vi "ClassProvidor_GoopOptionsDialog.vi"(8 "error in (no error)":errorcluster) -> (0 "error out":errorcluster)   [LabVIEW 2020]
uses:
  <resource>/Framework/Providers/Open_GDS/SubVIs/GOOP_HelpButton.ctl
  <resource>/Framework/Providers/Open_GDS/ClassProviders/Provider_EndevoGOOP300/EndevoProviderName.ctl
  <resource>/Framework/Providers/Open_GDS/ClassProviders/Provider_EndevoGOOP400/EndevoG4ProviderName.ctl
panel:
  in  "_InstallNewClassProvider":bool
  in  "_RemoveClassProvider":bool
  in  "_HelpGoopOption":T1
  in  "_AddClassProvider":bool
  out "Tab":enum32{"Select", "Add"}(tab)
  in  "_CurrentClassProvider":u16(ring) caption="Current Class provider to use:" items=["EndevoGOOP300", "Endevo LabVIEW Native", "EndevoGOOP400"]
  in  "_ConfigureCurrentClassProvider":bool
  out "ProductPicture":picture
  in  "_ProviderClassReaderPath":path caption="Provider Class Reader Path"
  in  "_ProviderClassWriterPath":path caption="Provider Class Writer Path"
  in  "_ProviderName":string caption="ProviderName"
  in  "_Cancel":bool
  in  "_OK":bool
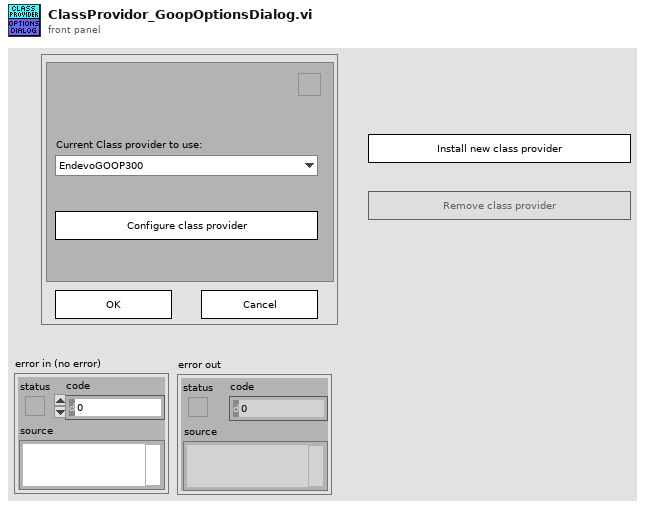
[diagram p1: front panel]
types:
  T1 = typedef "GOOP_HelpButton.ctl" = bool
  T2 = typedef "EndevoG4ProviderName.ctl" = enum16{"EndevoGOOP400"}
  T3 = typedef "EndevoProviderName.ctl" = enum16{"EndevoGOOP300"}
  T4 = cluster{"ClassProviders":string[], "Path":path, "ClassConfig":path}
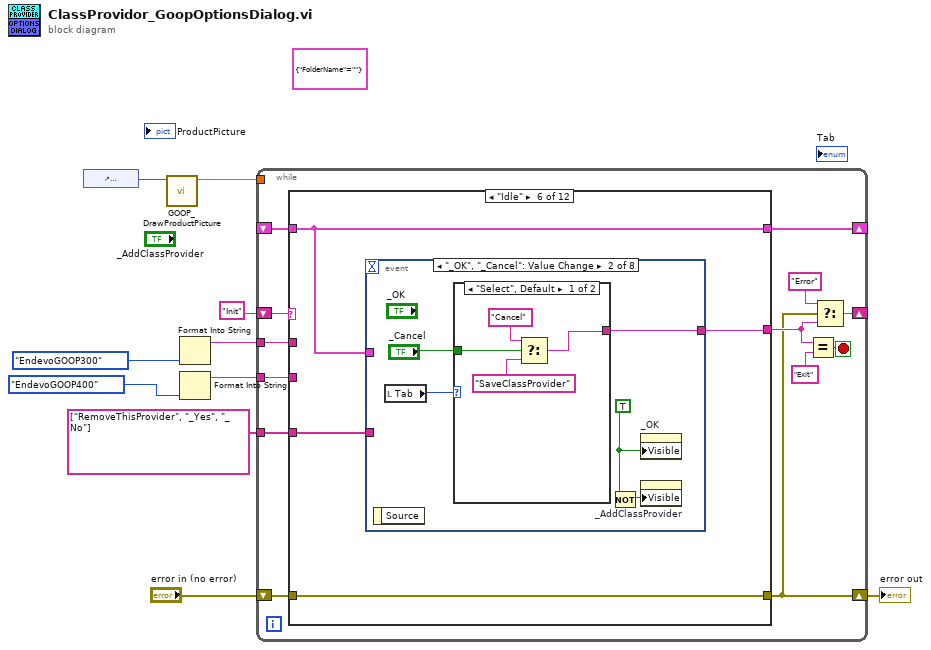
[diagram p0: block diagram]
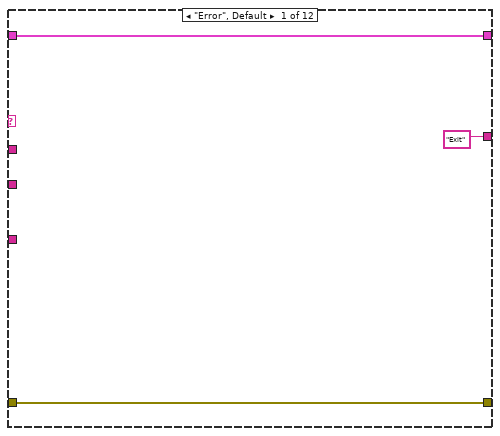
[diagram p2: hidden frame]
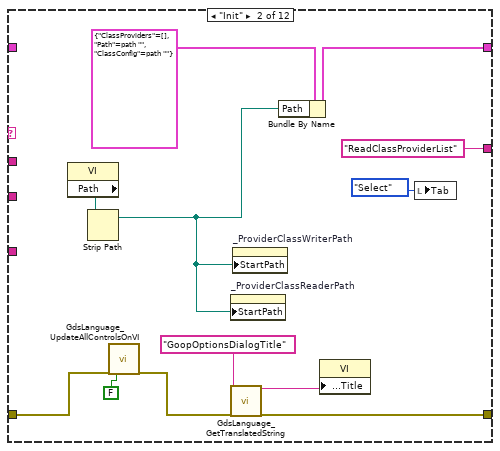
[diagram p3: hidden frame]
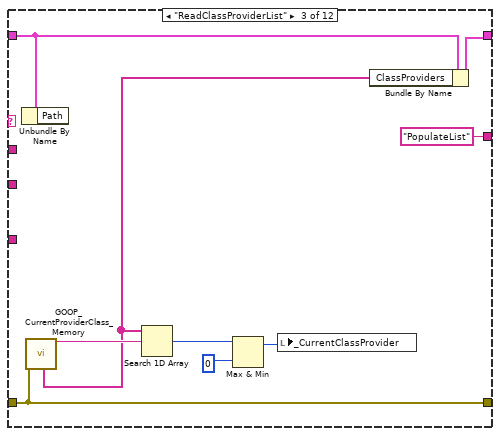
[diagram p4: hidden frame]
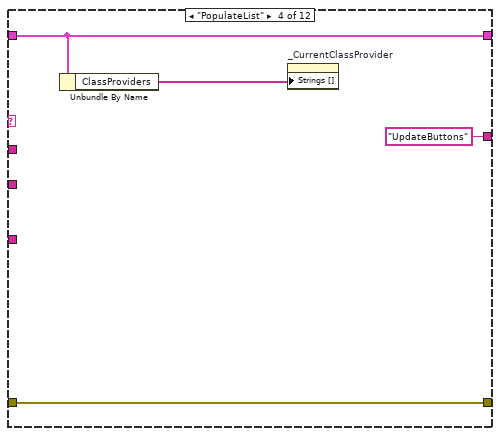
[diagram p5: hidden frame]
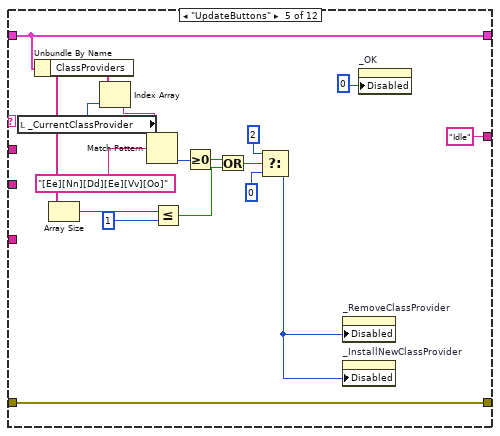
[diagram p6: hidden frame]
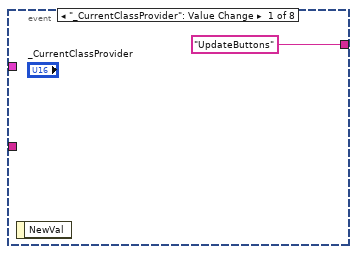
[diagram p7: hidden frame]
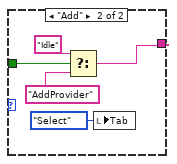
[diagram p8: hidden frame]
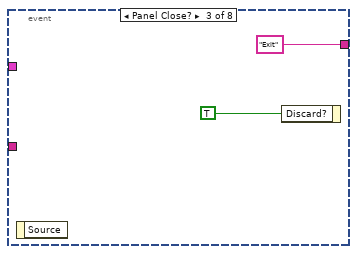
[diagram p9: hidden frame]
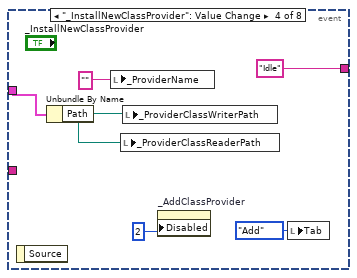
[diagram p10: hidden frame]
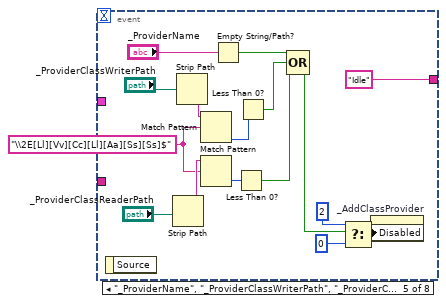
[diagram p11: hidden frame]
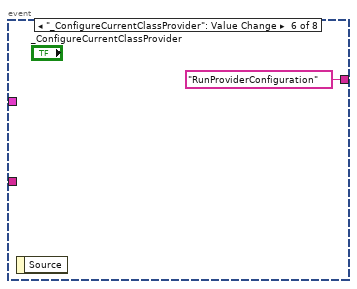
[diagram p12: hidden frame]
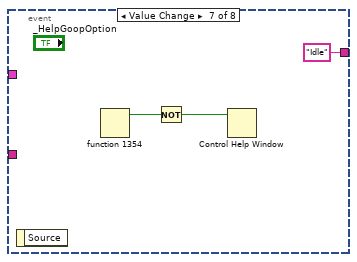
[diagram p13: hidden frame]
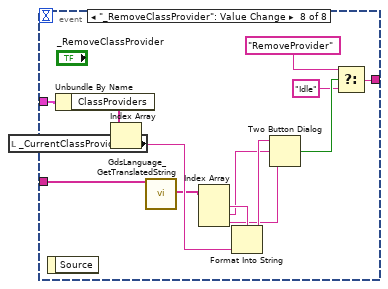
[diagram p14: hidden frame]
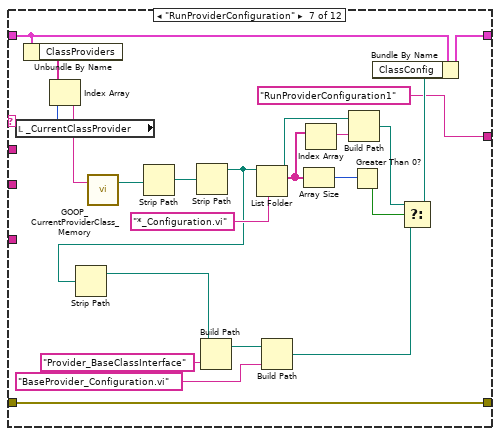
[diagram p15: hidden frame]
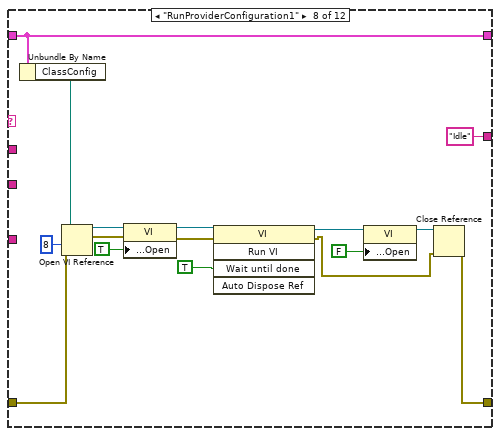
[diagram p16: hidden frame]
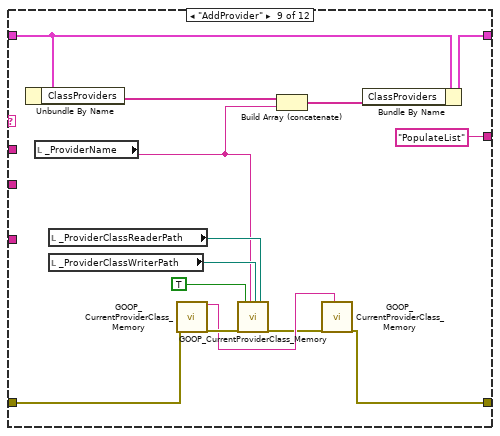
[diagram p17: hidden frame]
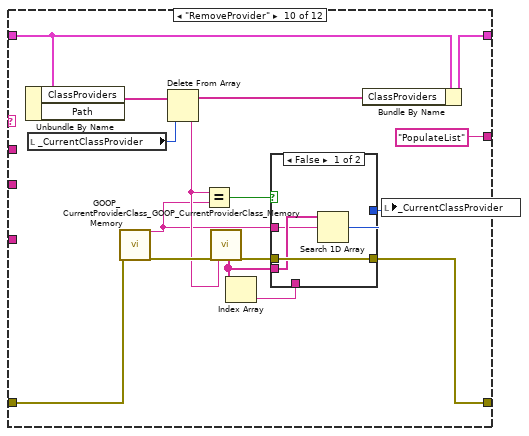
[diagram p18: hidden frame]
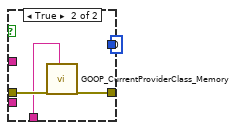
[diagram p19: hidden frame]
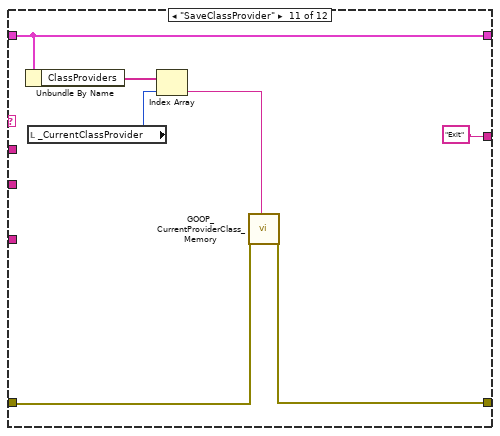
[diagram p20: hidden frame]
diagram:
  (unwired) cluster{"FolderName":string} {"FolderName"=""}
  n1 = control-ref of="ProductPicture"() -> (w2:refnum<vi>)
  n2 = call <resource>:"GOOP_DrawProductPicture.vi"("ProductPictureControl"=w2) -> ("Zoom Factor"=w1:sgl)  [unwired: 10 in]
  n3 = Format Into String(EndevoProviderName."EndevoGOOP300" ("ProviderName")) -> (resulting string=w4:string)  [unwired: 3 in, 1 out]
  n4 = Format Into String(EndevoG4ProviderName."EndevoGOOP400" ("ProviderName")) -> (resulting string=w3:string)  [unwired: 3 in, 1 out]
  n5 = while {
    shift-right: [w16] -> w8
    shift-left: "error in (no error)" -> [w23]
    shift-right: [w21] -> _
    shift-left: "Init" -> [w22]
    shift-right: [w15] -> _
    shift-left: _ -> [w14]
    tunnel: string[] ["RemoveThisProvider", "_Yes", "_No"] -> [w13]
    tunnel: w4 -> [w12]
    tunnel: w3 -> [w11]
    tunnel: w1 -> [_]
    stop <- w20 stop-if-true
    n6 = case shown="\"Idle\"" w22 {
      tunnel: w23 -> [w26 w31 w45 w48 w56 w71 w149 w167 w173 w192 w211 w214]
      tunnel: [w26 w28 w45 w48 w56 w71 w149 w165 w169 w186 w210 w214] -> w16
      tunnel: ["Exit" "ReadClassProviderList" "PopulateList" "UpdateButtons" "Idle" w72 "RunProviderConfiguration1" "Idle" ("f") "PopulateList" "PopulateList" "Exit" "Exit"] -> w17
      tunnel: [w24 w35 w46 w50 w58 w70 w147 w164 w182 w198 w213 w216] -> w15
      tunnel: w14 -> [w24 _ w42 w50 w58 w70 w148 w164 w181 w197 w213 w216]
      tunnel: w13 -> [_ _ _ _ _ w69 _ _ _ _ _ _]
      tunnel: w12 -> [_ _ _ _ _ _ _ _ _ _ _ _]
      tunnel: w11 -> [_ _ _ _ _ _ _ _ _ _ _ _]
      frame "Error", Default {
      }
      frame "Init" {
        n7 = property class="VI"() -> ("Path"=w34:path)  [unwired: 2 in, 2 out]
        n8 = Strip Path(path=w34) -> (stripped path=w33:path)  [unwired: 1 out]
        n9 = call <resource>:"GdsLanguage_UpdateAllControlsOnVI.vi"("error in (no error)"=w31, "CreateLanguageFile(Use this to create a languageFile)"=FALSE) -> ("error out"=w30:errorcluster)  [unwired: 16 in, 1 out]
        n10 = property on="_ProviderClassReaderPath" class="Path"("StartPath"=w33) -> ()  [unwired: 2 in, 2 out]
        n11 = call <resource>:"GdsLanguage_GetTranslatedString.vi"("StringID(s)"="GoopOptionsDialogTitle", "error in (no error)"=w30) -> ("FirstStringOut"=w27:string, "error out"=w28:errorcluster)  [unwired: 14 in, 2 out]
        n12 = property on="_ProviderClassWriterPath" class="Path"("StartPath"=w33) -> ()  [unwired: 2 in, 2 out]
        n13 = Bundle By Name(cluster=T4 {"ClassProviders"=[], "Path"=path "", "ClassConfig"=path ""}, "Path"=w33) -> (w35:T4)
        n14 = property class="VI"("Front Panel.Title"=w27) -> ()  [unwired: 2 in, 2 out]
        n15 = local write "Tab"(enum32{"Select", "Add"}."Select" ("Tab")) -> ()
      }
      frame "ReadClassProviderList" {
        n16 = Unbundle By Name(w42) -> ()  [unwired: 1 out]
        n17 = call <resource>:"GOOP_CurrentProviderClass_Memory.vi"("error in (no error)"=w45) -> ("AllClassProviders"=w43:string[], "ClassProviderName"=w44:string)  [unwired: 14 in, 3 out]
        n18 = Search 1D Array(1D array=w43, element=w44) -> (index of element=w41:i32)  [unwired: 1 in]
        n19 = Max & Min(x=w41, y=0 ("lower limit")) -> (max(x,y)=w39:i32)  [unwired: 1 out]
        n20 = local write "_CurrentClassProvider"(w39) -> ()
        n21 = Bundle By Name(cluster=w42, "ClassProviders"=w43) -> (w46:T4)
      }
      frame "PopulateList" {
        n22 = Unbundle By Name(w50) -> ("ClassProviders"=w49:string[])
        n23 = property on="_CurrentClassProvider" class="Ring (strict)"("Strings []"=w49) -> ()  [unwired: 2 in, 2 out]
      }
      frame "UpdateButtons" {
        n24 = local read "_CurrentClassProvider"() -> (w54:u16)
        n25 = Unbundle By Name(w58) -> ("ClassProviders"=w67:string[])
        n26 = Array Size(array=w67) -> (size(s)=w65:i32)
        n27 = Index Array(array=w67, index=w54) -> (element=w53:string)
        n28 = Match Pattern(string=w53, regular expression="[Ee][Nn][Dd][Ee][Vv][Oo]") -> (offset past match=w66:i32)  [unwired: 1 in, 3 out]
        n29 = Less Or Equal?(x=w65, y=1) -> (x <= y?=w62:bool)
        n30 = Greater Or Equal To 0?(x=w66) -> (x >= 0?=w63:bool)
        n31 = Or(x=w63, y=w62) -> (x .or. y?=w61:bool)
        n32 = Select(t=u8 2 ("Disabled"), s=w61, f=u8 0 ("Disabled")) -> (s? t:f=w52:u8)
        n33 = property on="_RemoveClassProvider" class="Bool"("Disabled"=w52) -> ()  [unwired: 2 in, 2 out]
        n34 = property on="_InstallNewClassProvider" class="Bool"("Disabled"=w52) -> ()  [unwired: 2 in, 2 out]
        n35 = property on="_OK" class="Bool"("Disabled"=u8 0) -> ()  [unwired: 2 in, 2 out]
      }
      frame "Idle" {
        n36 = event shown="[1] \"_OK\", \"_Cancel\": Value Change" {
          selector: _ -> [_ _ _ _ _ _ _ _]
          dyn-events: _ -> [_ _ _ _ _ _ _ _]
          timeout: _ -> [_ _ _ _ _ _ _ _]
          tunnel: ["UpdateButtons" w76 "Exit" "Idle" "Idle" "RunProviderConfiguration" ("f") "Idle" ("f") w123] -> w72
          tunnel: w70 -> [_ _ _ w91 _ _ _ w129]
          tunnel: w69 -> [_ _ _ _ _ _ _ w118]
          event "_CurrentClassProvider": Value Change {
            n37 = event-data() -> ()  [unwired: 1 in, 1 out]
          }
          event "_OK", "_Cancel": Value Change {
            w74 = TRUE ("Visible")
            n38 = event-data() -> ()  [unwired: 1 in, 1 out]
            n39 = local read "Tab"() -> (w78:enum32{"Select", "Add"})
            n40 = case shown="\"Select\", Default" w78 {
              tunnel: "_Cancel" -> [w82 w87]
              tunnel: [w81 w84] -> w76
              frame "Select", Default {
                n41 = Select(t="Cancel", s=w82, f="SaveClassProvider") -> (s? t:f=w81:string)
              }
              frame "Add" {
                n42 = Select(t="Idle", s=w87, f="AddProvider") -> (s? t:f=w84:string)
                n43 = local write "Tab"(enum32{"Select", "Add"}."Select" ("Tab")) -> ()
              }
            }
            n44 = Not(x=w74) -> (.not. x?=w75:bool)
            n45 = property on="_OK" class="Bool"("Visible"=w74) -> ()  [unwired: 2 in, 2 out]
            n46 = property on="_AddClassProvider" class="Bool"("Visible"=w75) -> ()  [unwired: 2 in, 2 out]
          }
          event Panel Close? {
            n47 = event-data() -> ()  [unwired: 1 in, 1 out]
            n48 = event-data("Discard?"=TRUE) -> ()  [unwired: 1 in, 1 out]
          }
          event "_InstallNewClassProvider": Value Change {
            n49 = event-data() -> ()  [unwired: 1 in, 1 out]
            n50 = Unbundle By Name(w91) -> ("Path"=w90:path)
            n51 = local write "_ProviderName"("" ("Provider folder name:")) -> ()
            n52 = local write "_ProviderClassReaderPath"(w90) -> ()
            n53 = local write "_ProviderClassWriterPath"(w90) -> ()
            n54 = property on="_AddClassProvider" class="Bool"("Disabled"=u8 2) -> ()  [unwired: 2 in, 2 out]
            n55 = local write "Tab"(enum32{"Select", "Add"}."Add" ("Tab")) -> ()
          }
          event "_ProviderName", "_ProviderClassWriterPath", "_ProviderClassReaderPath": Value Change {
            w98 = "\\2E[Ll][Vv][Cc][Ll][Aa][Ss][Ss]$" ("regular expression")
            n56 = event-data() -> ()  [unwired: 1 in, 1 out]
            n57 = Strip Path(path="_ProviderClassReaderPath") -> (name=w99:string)  [unwired: 1 out]
            n58 = Strip Path(path="_ProviderClassWriterPath") -> (name=w103:string)  [unwired: 1 out]
            n59 = Match Pattern(string=w103, regular expression=w98) -> (offset past match=w102:i32)  [unwired: 1 in, 3 out]
            n60 = Match Pattern(string=w99, regular expression=w98) -> (offset past match=w97:i32)  [unwired: 1 in, 3 out]
            n61 = Empty String/Path?(string/path="_ProviderName") -> (empty?=w106:bool)
            n62 = Less Than 0?(x=w97) -> (x < 0?=w96:bool)
            n63 = Less Than 0?(x=w102) -> (x < 0?=w101:bool)
            n64 = Compound Arithmetic op=OR(w106, w101, w96) -> (w105:bool)
            n65 = Select(t=u8 2 ("Disabled"), s=w105, f=u8 0) -> (s? t:f=w109:u8)
            n66 = property on="_AddClassProvider" class="Bool"("Disabled"=w109) -> ()  [unwired: 2 in, 2 out]
          }
          event "_ConfigureCurrentClassProvider": Value Change {
            n67 = event-data() -> ()  [unwired: 1 in, 1 out]
          }
          event Value Change {
            n68 = event-data() -> ()  [unwired: 1 in, 1 out]
            n69 = fn#1354() -> (1:w115:bool)  [unwired: 1 out]
            n70 = Not(x=w115) -> (.not. x?=w114:bool)
            n71 = Control Help Window(1:w114) -> ()  [unwired: 1 in]
          }
          event "_RemoveClassProvider": Value Change {
            n72 = local read "_CurrentClassProvider"() -> (w127:u16)
            n73 = event-data() -> ()  [unwired: 1 in, 1 out]
            n74 = Unbundle By Name(w129) -> ("ClassProviders"=w128:string[])
            n75 = Index Array(array=w128, index=w127) -> (element=w121:string)
            n76 = call <resource>:"GdsLanguage_GetTranslatedString.vi"("StringID(s)"=w118) -> ("StringsOut"=w120:string[])  [unwired: 15 in, 3 out]
            n77 = Index Array(array=w120) -> (element #1=w119:string, element #2=w117:string, element #3=w116:string)  [unwired: 3 in]
            n78 = Format Into String(format string=w119, w121) -> (resulting string=w126:string)  [unwired: 2 in, 1 out]
            n79 = Two Button Dialog(message=w126, 1:w116, 2:w117) -> (T button?=w125:bool)
            n80 = Select(t="RemoveProvider", s=w125, f="Idle") -> (s? t:f=w123:string)
          }
        }
      }
      frame "RunProviderConfiguration" {
        n81 = local read "_CurrentClassProvider"() -> (w151:u16)
        n82 = Unbundle By Name(w148) -> ("ClassProviders"=w152:string[])
        n83 = Index Array(array=w152, index=w151) -> (element=w150:string)
        n84 = call <resource>:"GOOP_CurrentProviderClass_Memory.vi"("GetThisClassProvidersPaths(Returns the default providor if not wired)"=w150) -> ("ClassProviderClassWriterPath"=w141:path)  [unwired: 14 in, 4 out]
        n85 = Strip Path(path=w141) -> (stripped path=w140:path)  [unwired: 1 out]
        n86 = Strip Path(path=w140) -> (stripped path=w131:path)  [unwired: 1 out]
        n87 = Strip Path(path=w131) -> (stripped path=w130:path)  [unwired: 1 out]
        n88 = Build Path(base path=w130, name or relative path="Provider_BaseClassInterface") -> (appended path=w143:path)
        n89 = List Folder(path=w131, pattern="*_Configuration.vi" ("name or relative path")) -> (path out=w133:path, filenames=w135:string[])  [unwired: 2 in, 2 out]
        n90 = Build Path(base path=w143, name or relative path="BaseProvider_Configuration.vi") -> (appended path=w137:path)
        n91 = Array Size(array=w135) -> (size(s)=w138:i32)
        n92 = Index Array(array=w135) -> (element=w134:string)  [unwired: 1 in]
        n93 = Build Path(base path=w133, name or relative path=w134) -> (appended path=w132:path)
        n94 = Greater Than 0?(x=w138) -> (x > 0?=w136:bool)
        n95 = Select(t=w132, s=w136, f=w137) -> (s? t:f=w146:path)
        n96 = Bundle By Name(cluster=w148, "ClassConfig"=w146) -> (w147:T4)
      }
      frame "RunProviderConfiguration1" {
        n97 = Unbundle By Name(w164) -> ("ClassConfig"=w168:path)
        n98 = Open VI Reference(vi path=w168, options=8, error in (no error)=w167) -> (vi reference=w161:refnum<vi>, error out=w162:errorcluster)  [unwired: 3 in]
        n99 = property class="VI"(reference=w161, error in=w162, "Front Panel.Open"=TRUE ("Front Panel Window:Open")) -> (reference out=w160:refnum<vi>, error out=w159:errorcluster)
        n100 = invoke class="VI" method="Run VI"(reference=w160, error in=w159, "Wait until done"=TRUE ("Wait Until Done")) -> (reference out=w156:refnum<vi>, error out=w154:errorcluster)  [unwired: 2 in, 3 out]
        n101 = property class="VI"(reference=w156, "Front Panel.Open"=FALSE ("Front Panel Window:Open")) -> (reference out=w155:refnum<vi>)  [unwired: 1 in, 1 out]
        n102 = Close Reference(reference=w155, error in (no error)=w154) -> (error out=w165:errorcluster)
      }
      frame "AddProvider" {
        n103 = Unbundle By Name(w181) -> ("ClassProviders"=w180:string[])
        n104 = local read "_ProviderName"() -> (w175:string)
        n105 = local read "_ProviderClassReaderPath"() -> (w176:path)
        n106 = local read "_ProviderClassWriterPath"() -> (w177:path)
        n107 = call <resource>:"GOOP_CurrentProviderClass_Memory.vi"("error in (no error)"=w173) -> ("ClassProviderName"=w171:string, "error out"=w172:errorcluster)  [unwired: 14 in, 3 out]
        n108 = call <resource>:"GOOP_CurrentProviderClass_Memory.vi"("error in (no error)"=w172, "Don't Set just update"=TRUE, "SetDefaultClassProvider(Ignored if not wired)"=w175, "ClassProviderClassWriterPath(Used if not empty)"=w177, "ClassProviderClassReaderPath(Used if not empty)"=w176) -> ("error out"=w170:errorcluster)  [unwired: 10 in, 4 out]
        n109 = Build Array (concatenate)(w180, w175) -> (w179:string[])
        n110 = call <resource>:"GOOP_CurrentProviderClass_Memory.vi"("error in (no error)"=w170, "SetDefaultClassProvider(Ignored if not wired)"=w171) -> ("error out"=w169:errorcluster)  [unwired: 13 in, 4 out]
        n111 = Bundle By Name(cluster=w181, "ClassProviders"=w179) -> (w182:T4)
      }
      frame "RemoveProvider" {
        n112 = Unbundle By Name(w197) -> ("ClassProviders"=w195:string[])  [unwired: 1 out]
        n113 = local read "_CurrentClassProvider"() -> (w193:u16)
        n114 = call <resource>:"GOOP_CurrentProviderClass_Memory.vi"("error in (no error)"=w192) -> ("ClassProviderName"=w183:string, "error out"=w191:errorcluster)  [unwired: 14 in, 3 out]
        n115 = Delete From Array(array=w195, index=w193) -> (deleted portion=w190:string, array with subset deleted=w194:string[])  [unwired: 1 in]
        n116 = Equal?(x=w190, y=w183) -> (x = y?=w189:bool)
        n117 = call <resource>:"GOOP_CurrentProviderClass_Memory.vi"("error in (no error)"=w191, "RemoveThisClassProvidersPaths(Ignored if not wired)"=w190) -> ("AllClassProviders"=w184:string[], "error out"=w188:errorcluster)  [unwired: 13 in, 3 out]
        n118 = Index Array(array=w184) -> (element=w187:string)  [unwired: 1 in]
        n119 = case shown="False" w189 {
          tunnel: w188 -> [w202 w206]
          tunnel: w187 -> [_ w205]
          tunnel: [w202 w204] -> w186
          tunnel: [w199 u16 0 ("x")] -> w185
          tunnel: w184 -> [w201 _]
          tunnel: w183 -> [w200 _]
          frame False {
            n120 = Search 1D Array(1D array=w201, element=w200) -> (index of element=w199:i32)  [unwired: 1 in]
          }
          frame True {
            n121 = call <resource>:"GOOP_CurrentProviderClass_Memory.vi"("error in (no error)"=w206, "SetDefaultClassProvider(Ignored if not wired)"=w205) -> ("error out"=w204:errorcluster)  [unwired: 13 in, 4 out]
          }
        }
        n122 = Bundle By Name(cluster=w197, "ClassProviders"=w194) -> (w198:T4)
        n123 = local write "_CurrentClassProvider"(w185) -> ()
      }
      frame "SaveClassProvider" {
        n124 = Unbundle By Name(w213) -> ("ClassProviders"=w209:string[])
        n125 = local read "_CurrentClassProvider"() -> (w208:u16)
        n126 = Index Array(array=w209, index=w208) -> (element=w207:string)
        n127 = call <resource>:"GOOP_CurrentProviderClass_Memory.vi"("error in (no error)"=w211, "SetDefaultClassProvider(Ignored if not wired)"=w207) -> ("error out"=w210:errorcluster)  [unwired: 13 in, 4 out]
      }
      frame "Cancel" {
      }
    }
    n128 = Equal?(x=w17, y="Exit") -> (x = y?=w20:bool)
    n129 = Select(t="Error", s=w16, f=w17) -> (s? t:f=w21:string)
  }
  "error out" <- w8
